vi "Create_LogTimebase.vi"(5 "Samples per Decade":i32=128, 6 "end":dbl=1.0 format="%0.2f", 7 "start":dbl format="%.3ps") -> (3 "Log Ramp Pattern":dbl[](array[numeric]))   [LabVIEW 2014]
uses:
  <vilib>/Analysis/1siggen.llb/Ramp Pattern by Samples.vi
  <vilib>/Analysis/NI_AALBase.lvlib
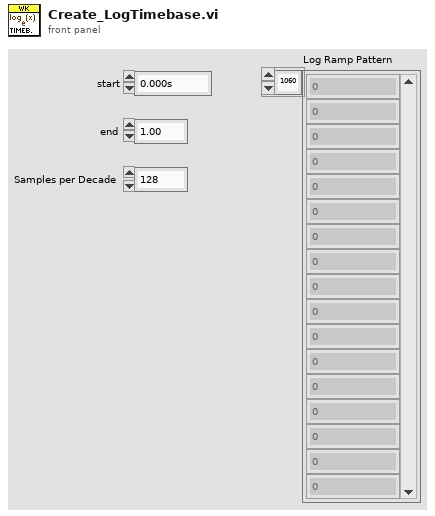
[diagram p1: front panel]
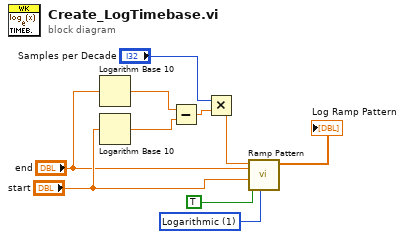
[diagram p0: block diagram]
diagram:
  w10 = u16 1 items=["Linear", "Logarithmic"] ("type")
  n1 = Logarithm Base 10(1:"end") -> (0:w1:dbl)
  n2 = Logarithm Base 10(1:"start") -> (0:w2:dbl)
  n3 = Subtract(x=w1, y=w2) -> (x-y=w5:dbl)
  n4 = Multiply(x="Samples per Decade", y=w5) -> (x*y=w3:dbl)
  n5 = call-poly <vilib>:"Ramp Pattern.vi"("type"=w10, "exclude end?"=TRUE, "start"="start", "end"="end", "samples"=w3) -> ("Ramp Pattern"=→"Log Ramp Pattern":dbl[])  [unwired: 5 in, 1 out]
